vi "Software heartbeat.vi"() -> (3 "SW Heartbeat":bool)   [LabVIEW 2017]
panel:
  out "Boolean 2":bool
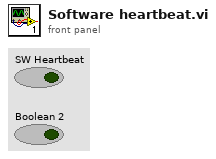
[diagram p1: front panel]
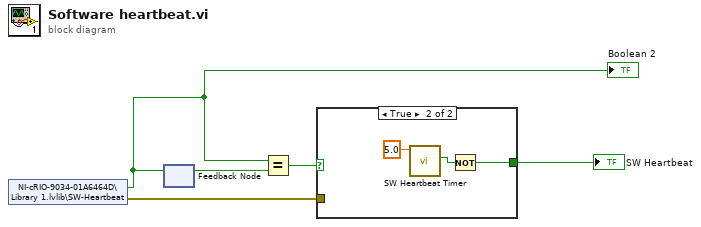
[diagram p0: block diagram]
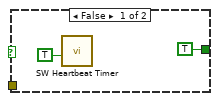
[diagram p2: hidden frame]
diagram:
  n1 = shared-variable "NI-cRIO-9034-01A6464D\\Library 1.lvlib\\SW-Heartbeat"() -> (w2:bool, error out=w5:errorcluster)  [unwired: 1 in]
  "Boolean 2" <- w2
  n2 = feedback #1() -> (w1:bool)  [unwired: 1 in]
  n3 = feedback-in #1(w2) -> ()
  n4 = Equal?(x=w2, y=w1) -> (x = y?=w3:bool)
  n5 = case shown="True" w3 {
    tunnel: [TRUE w8] -> w4
    tunnel: w5 -> [_ _]
    frame False {
      n6 = call "SW Heartbeat Timer.vi"("Reset"=TRUE) -> ()  [unwired: 8 in, 3 out]
    }
    frame True {
      n7 = call "SW Heartbeat Timer.vi"("Target Time"=5.0) -> ("Time Elapsed"=w9:bool)  [unwired: 8 in, 2 out]
      n8 = Not(x=w9) -> (.not. x?=w8:bool)
    }
  }
  "SW Heartbeat" <- w4
